vi "Periodic Tasks.vi"(8 "error in":errorcluster) -> (0 "error out":errorcluster)   [LabVIEW 2018]
doc: "This VI runs in parallel to other tasks. It can contain as many user-defined periodic loops as you need. These can carry out PID or other sorts of timed response."
uses:
  TypeDefs/Teleop Data Cluster.ctl
  TypeDefs/typedef_enum_TT_Input.ctl
  TypeDefs/typedef_enum_TT_Output.ctl
panel:
  in  "TeleOp Data Cluster":T1
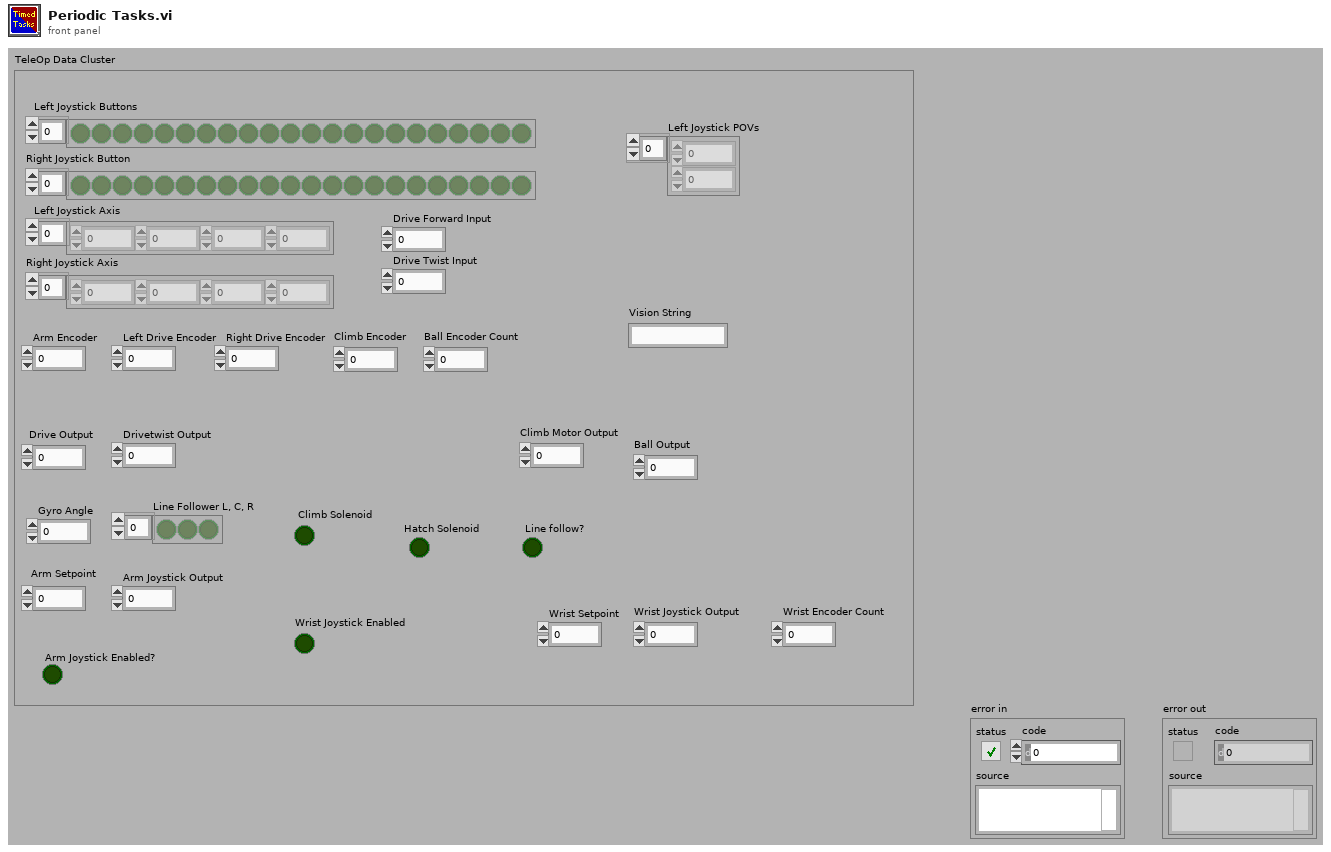
[diagram p1: front panel]
types:
  T1 = typedef "Teleop Data Cluster.ctl" = cluster{"Drive Forward Input ":dbl, "Drive Twist Input":dbl, "Drive Output":dbl, "Drivetwist Output":dbl, "Left Joystick Buttons":bool[], "Left Joystick Axis":dbl[], "Right Joystick Axis":dbl[], "Right Joystick Button":bool[], "Arm Encoder":dbl, "Left Drive Encoder":dbl, "Right Drive Encoder":dbl, "Gyro Angle ":dbl, "Arm Joystick Output  ":dbl, "Line Follower L, C, R ":bool[], "Line follow?":bool, " Climb Solenoid":bool, "Wrist Encoder Count":dbl, "Wrist Joystick Output":dbl, "Ball Encoder Count":dbl, "Ball Output":dbl, "Climb Encoder":dbl, "Climb Motor Output":dbl, " Hatch Solenoid":bool, "Arm Setpoint ":dbl, "Wrist Setpoint ":dbl, "Arm Joystick Enabled?":bool, "Wrist Joystick Enabled":bool, "Vision String":string, "Left Joystick POVs":i16[]}
  T2 = typedef "typedef_enum_TT_Output.ctl" = enum16{"Wait", "Output", "Notification"}
  T3 = typedef "typedef_enum_TT_Input.ctl" = enum16{"Read Values", "Write_Notifier", "Wait"}
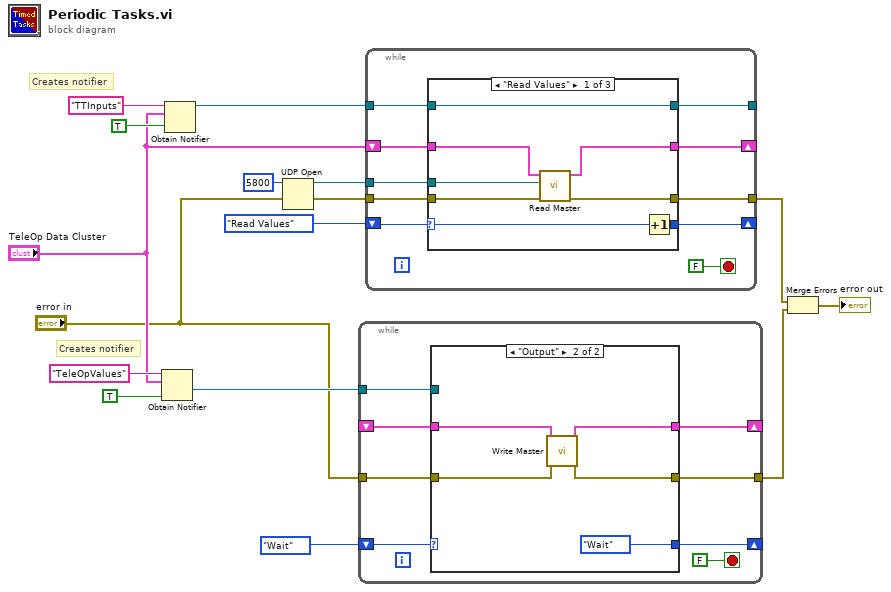
[diagram p0: block diagram]
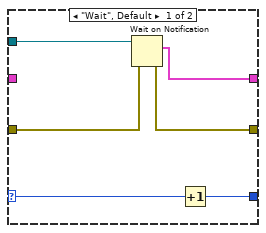
[diagram p2: hidden frame]
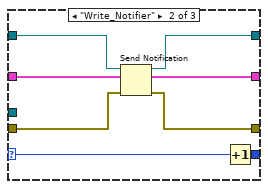
[diagram p3: hidden frame]
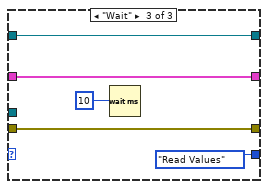
[diagram p4: hidden frame]
diagram:
  # "Creates notifier"
  # "Creates notifier"
  n1 = Obtain Notifier(name (unnamed)="TeleOpValues", notification data type="TeleOp Data Cluster", create if not found? (T)=TRUE) -> (notifier out=w9:refnum<notifier>)  [unwired: 1 in, 2 out]
  n2 = Obtain Notifier(name (unnamed)="TTInputs", notification data type="TeleOp Data Cluster", create if not found? (T)=TRUE) -> (notifier out=w12:refnum<notifier>)  [unwired: 1 in, 2 out]
  n3 = UDP Open(11:u16 5800 ("port")) -> (port=w2:refnum<k16>)  [unwired: 4 in, 2 out]
  n4 = while {
    shift-right: [w18] -> _
    shift-left: typedef_enum_TT_Output."Wait" ("Enum") -> [w23]
    tunnel: w9 -> [w22]
    shift-right: [w20] -> _
    shift-left: _ -> [w19]
    tunnel: "error in" -> [w17]
    tunnel: [w16] -> w5
    stop <- FALSE stop-if-true
    n5 = case shown="\"Output\"" w23 {
      selector: w23 -> [w24 _]
      tunnel: w22 -> [w28 _]
      tunnel: [w27 w31] -> w20
      tunnel: w19 -> [_ w30]
      tunnel: [w29 typedef_enum_TT_Output."Wait"] -> w18
      tunnel: w17 -> [w26 w32]
      tunnel: [w25 w33] -> w16
      frame "Wait", Default {
        n6 = Wait on Notification(notifier=w28, error in (no error)=w26) -> (notification=w27:T1, error out=w25:errorcluster)  [unwired: 2 in, 2 out]
        n7 = Increment(x=w24) -> (x+1=w29:T2)
      }
      frame "Output" {
        n8 = call "Write Master.vi"("error in"=w32, "TeleOp Data in"=w30) -> ("error out"=w33:errorcluster, "TeleOp Data out"=w31:T1)  [unwired: 8 in]
      }
    }
  }
  n9 = while {
    shift-right: [w38] -> _
    shift-left: typedef_enum_TT_Input."Read Values" ("Enum") -> [w44]
    tunnel: w12 -> [w41]
    shift-right: [w42] -> _
    shift-left: "TeleOp Data Cluster" -> [w43]
    tunnel: [w40] -> _
    tunnel: "error in" -> [w37]
    tunnel: [w36] -> w6
    tunnel: w2 -> [w35]
    stop <- FALSE stop-if-true
    n10 = case shown="\"Read Values\"" w44 {
      selector: w44 -> [w51 w56 _]
      tunnel: w43 -> [w49 w57 w63]
      tunnel: [w48 w57 w63] -> w42
      tunnel: w41 -> [w52 w59 w62]
      tunnel: [w52 w58 w62] -> w40
      tunnel: [w50 w55 typedef_enum_TT_Input."Read Values"] -> w38
      tunnel: w37 -> [w46 w54 w60]
      tunnel: [w47 w53 w60] -> w36
      tunnel: w35 -> [w45 _ _]
      frame "Read Values" {
        n11 = call "Read Master.vi"("error in"=w46, "connection ID"=w45, "TeleOp Data in"=w49) -> ("error out"=w47:errorcluster, "TeleOp Data out"=w48:T1)  [unwired: 7 in]
        n12 = Increment(x=w51) -> (x+1=w50:T3)
      }
      frame "Write_Notifier" {
        n13 = Send Notification(notification=w57, notifier=w59, error in (no error)=w54) -> (notifier out=w58:refnum<notifier>, error out=w53:errorcluster)
        n14 = Increment(x=w56) -> (x+1=w55:T3)
      }
      frame "Wait" {
        n15 = Wait (ms)(milliseconds to wait=u32 10) -> ()  [unwired: 1 out]
      }
    }
  }
  n16 = Merge Errors(w6, w5) -> (→"error out":errorcluster)
